vi "GetInstance.vi"(8 "error in (no error)":errorcluster, 11 "Konvolucio MCAN120803 Adapter Class in":refnum<class "Konvolucio MCAN120803 Adapter Class.lvclass">) -> (0 "error out":errorcluster, 2 "Values":string[](array[string]), 3 "Konvolucio MCAN120803 Adapter Class out":refnum<class "Konvolucio MCAN120803 Adapter Class.lvclass">)   [LabVIEW 2011, in "Konvolucio MCAN120803 Adapter Class.lvclass"]
uses:
  Konvolucio MCAN120803 Adapter Class.lvclass
  <instrlib>/Konvolucio MCAN120803/Konvolucio MCAN120803.lvlib
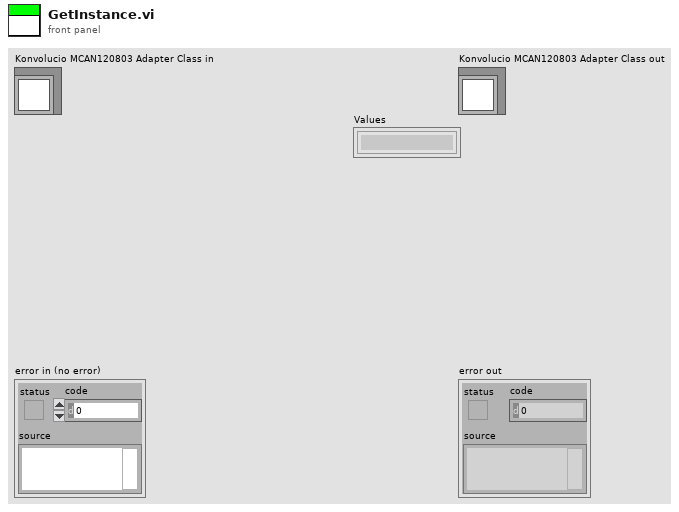
[diagram p1: front panel]
types:
  T1 = typedef "Konvolucio MCAN120803.lvlib/AdapterItemType.ctl" = cluster{"Name":string, "DeviceDescription":string, "SerialNumber":string, "InUse":bool, "Handle":refnum<k24>}
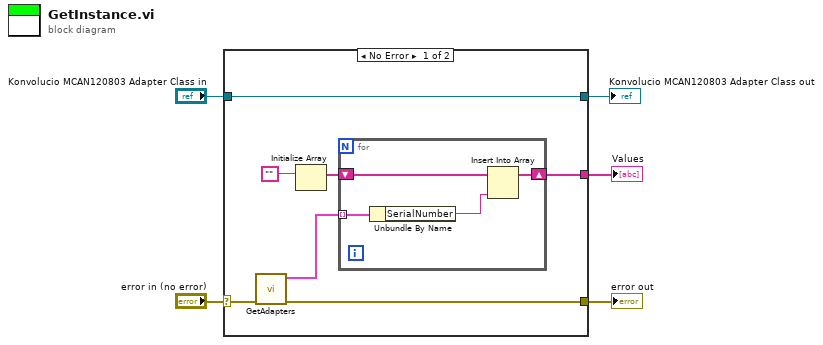
[diagram p0: block diagram]
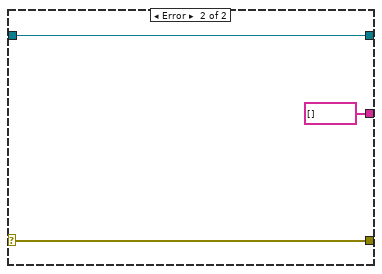
[diagram p2: hidden frame]
diagram:
  n1 = case shown="No Error" "error in (no error)" {
    selector: "error in (no error)" -> [w8 w19]
    tunnel: [w9 string[] []] -> w4
    tunnel: [w7 w19] -> w3
    tunnel: [w6 w18] -> w2
    tunnel: "Konvolucio MCAN120803 Adapter Class in" -> [w6 w18]
    frame No Error {
      n2 = call <instrlib>:"GetAdapters.vi"("error in"=w8) -> ("error out"=w7:errorcluster, "AdaptersOut"=w12:T1[])  [unwired: 9 in]
      n3 = Initialize Array("") -> (w10:string[])  [unwired: 1 in]
      n4 = for {
        tunnel: w12 -> [w16] mode=indexing
        shift-right: [w14] -> w9
        shift-left: w10 -> [w15]
        n5 = Unbundle By Name(w16) -> ("SerialNumber"=w13:string)
        n6 = Insert Into Array(array=w15, new element=w13) -> (w14:string[])  [unwired: 1 in]
      }
    }
    frame Error {
    }
  }
  "error out" <- w3
  "Konvolucio MCAN120803 Adapter Class out" <- w2
  "Values" <- w4
